vi "set delay mode.vi"(6 "jumplengthlimit":u16, 7 "minjumpdelay":u16, 8 "error in (no error)":errorcluster, 9 "edgelevel":u16, 10 "directmove3d":u16, 11 "varpoly":u16) -> (0 "error out":errorcluster)   [LabVIEW 2015, in "SCANalone4x64.lvlib"]
doc: "__declspec(dllimport) void __stdcall set_delay_mode(unsigned short varpoly, unsigned short directmove3d, unsigned short edgelevel, unsigned short minjumpdelay, unsigned short jumplengthlimit);"
uses:
  <userlib>/SCANalone4x64/SCANalone4x64.lvlib
  <userlib>/SCANalone4x64/SCANalone4x64.dll
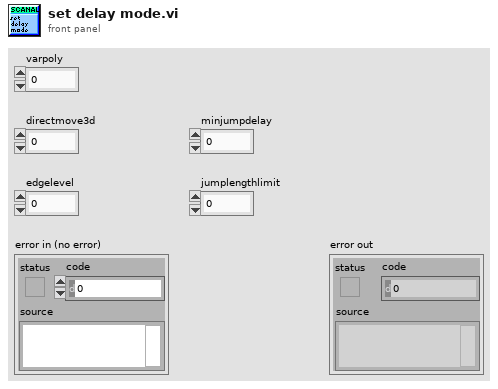
[diagram p1: front panel]
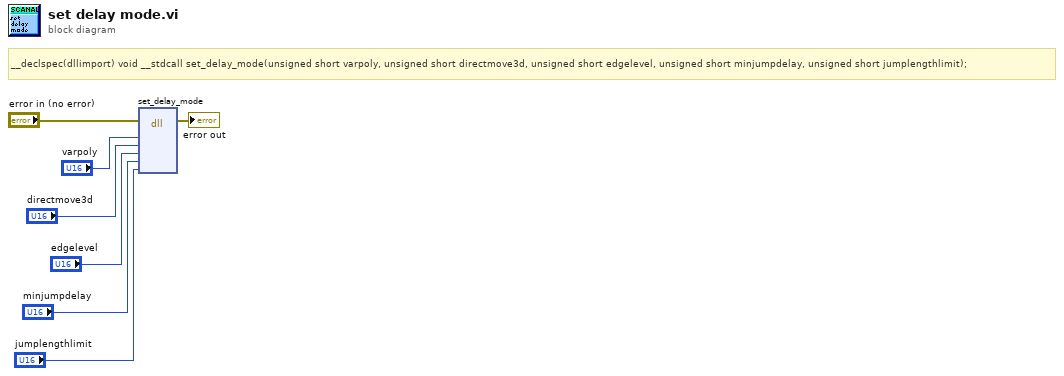
[diagram p0: block diagram]
diagram:
  # "__declspec(dllimport) void __stdcall set_delay_mode(unsigned short varpoly, unsigned short directmove3d, unsigned short edgelevel, unsigned short minjumpdelay, unsigned short jumplengthlimit);"
  n1 = dll-call lib="C:/Program Files/National Instruments/LabVIEW 2015/user.lib/SCANalone4x64/SCANalone4x64.*" fn="set_delay_mode"(error in="error in (no error)", "varpoly"="varpoly", "directmove3d"="directmove3d", "edgelevel"="edgelevel", "minjumpdelay"="minjumpdelay", "jumplengthlimit"="jumplengthlimit") -> (error out=→"error out":errorcluster)  [unwired: 8 in, 1 out]
